vi "Send M1M3 State Event.vi"(8 "error in (no error)":errorcluster, 10 "M1M3 Support State":T1, 11 "M1M3 Support Events in":refnum<class "M1M3 Support Events.lvclass">) -> (0 "error out":errorcluster, 3 "M1M3 Support Events out":refnum<class "M1M3 Support Events.lvclass">)   [LabVIEW 2016, in "M1M3 Support Events.lvclass"]
uses:
  M1M3 Support Events.lvclass
  Typedefs/StateTypes.ctl
  M1M3 Support Events.lvclass/M1M3 Support Events.ctl
  Typedefs/M1M3SupportEUI_TypeDefs.lvlib
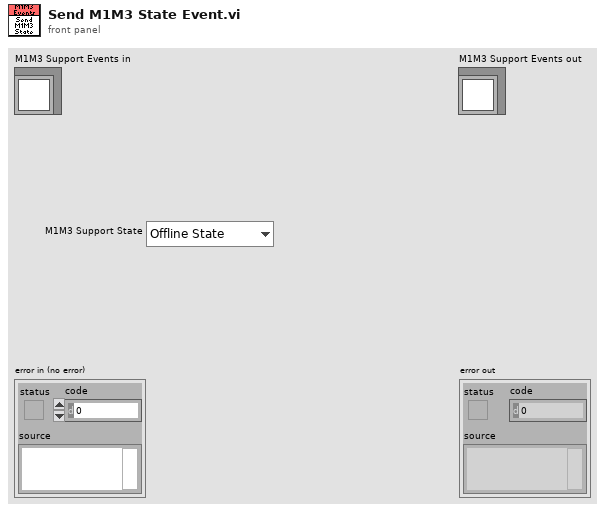
[diagram p1: front panel]
types:
  T1 = typedef "M1M3SupportEUI_TypeDefs.lvlib/StateTypes.ctl" = enum16{"Offline State", "Fault State", "Standby State", "Disabled State", "Enabled State", "Wait For User Input State", "Test Actuator State"}
  T2 = typedef "M1M3SupportEUI_TypeDefs.lvlib/M1M3 Support Events.ctl" = cluster{"M1M3 Support State":refnum<user-event>, "Inclinometer  Data":refnum<user-event>, "IMS Data":refnum<user-event>}
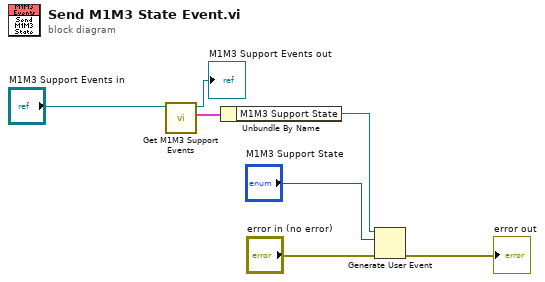
[diagram p0: block diagram]
diagram:
  n1 = call "Get M1M3 Support Events.vi"("M1M3 Support Events in"="M1M3 Support Events in") -> ("M1M3 Support Events"=w7:T2, "M1M3 Support Events out"=→"M1M3 Support Events out":refnum<class "M1M3 Support Events.lvclass">)  [unwired: 9 in]
  n2 = Unbundle By Name(w7) -> ("M1M3 Support State"=w6:refnum<user-event>)
  n3 = Generate User Event(user event=w6, event data cluster="M1M3 Support State", error in="error in (no error)") -> (error out=→"error out":errorcluster)  [unwired: 1 in, 1 out]
